vi "array to operate on concatenate and append mode.vi"() -> ()   [LabVIEW 2012]
panel:
  in  "Tab Control":enum32{"Concatenate Mode", "Append mode"}(tab)
  in  "Array 5":dbl[](array[numeric])
  in  "Array 4":dbl[](array[numeric])
  in  "Array 6":dbl[](array[numeric])
  in  "array":dbl
  out "Concatenated array":dbl[](array[numeric])
  in  "Array 7":dbl[](array[numeric])
  in  "Array 8":dbl[](array[numeric])
  in  "Array 9":dbl[](array[numeric])
  out "appended array":dbl[][](array[numeric])
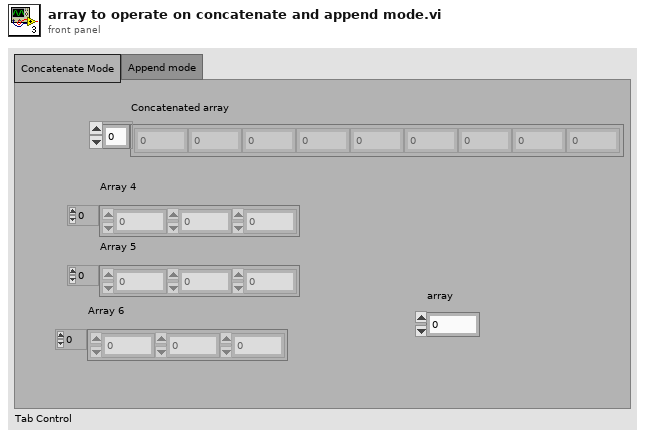
[diagram p1: front panel]
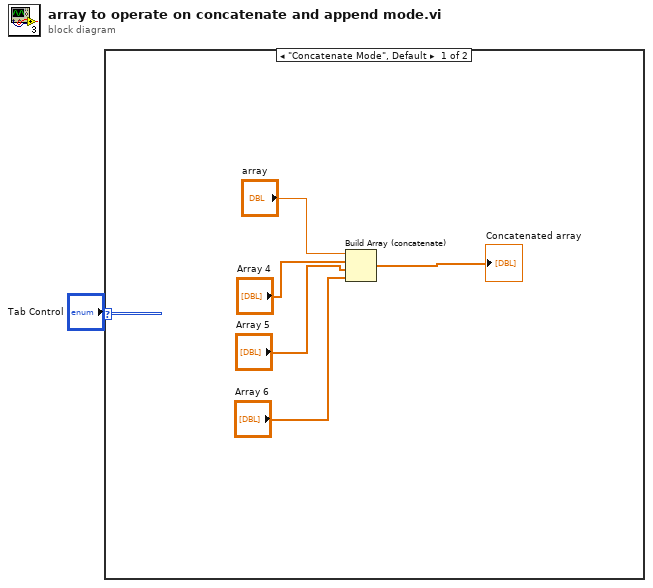
[diagram p0: block diagram]
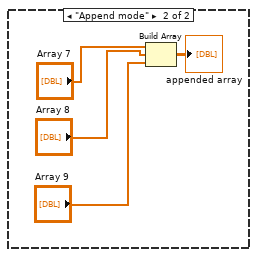
[diagram p2: hidden frame]
diagram:
  n1 = case shown="\"Concatenate Mode\", Default" "Tab Control" {
    frame "Concatenate Mode", Default {
      n2 = Build Array (concatenate)("array", "Array 4", "Array 5", "Array 6") -> (→"Concatenated array":dbl[])
    }
    frame "Append mode" {
      n3 = Build Array("Array 7", "Array 8", "Array 9") -> (→"appended array":dbl[][])
    }
  }
